vi "[X] = X0 [DBL].vi"(1 "Tolerance (1E-6)":dbl=1e-06, 7 "X":dbl[](array[numeric]) format="%#_9g") -> (8 "All Identical?":bool)   [LabVIEW 2021, in "Comparison.lvlib"]
uses:
  Comparison.lvlib
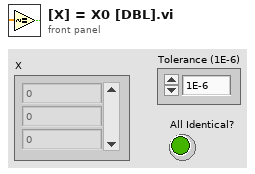
[diagram p1: front panel]
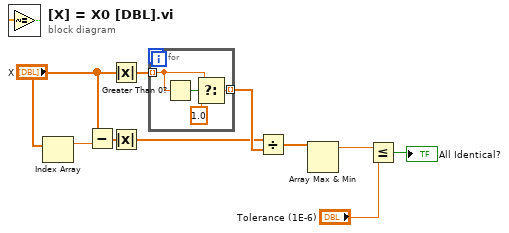
[diagram p0: block diagram]
diagram:
  n1 = Index Array(array="X") -> (element=w1:dbl)  [unwired: 1 in]
  n2 = Subtract(x="X", y=w1) -> (x-y=w8:dbl[])
  n3 = Absolute Value(x="X") -> (abs(x)=w7:dbl[])
  n4 = Absolute Value(x=w8) -> (abs(x)=w5:dbl[])
  n5 = for {
    tunnel: w7 -> [w13] mode=indexing
    tunnel: [w11] -> w6 mode=indexing
    n6 = Greater Than 0?(x=w13) -> (x > 0?=w14:bool)
    n7 = Select(t=w13, s=w14, f=1.0) -> (s? t:f=w11:dbl)
  }
  n8 = Divide(x=w5, y=w6) -> (x/y=w4:dbl[])
  n9 = Array Max & Min(array=w4) -> (max value=w10:dbl)  [unwired: 3 out]
  n10 = Less Or Equal?(x=w10, y="Tolerance (1E-6)") -> (x <= y?=→"All Identical?":bool)
